vi "Create AI Channel.vi"(8 "error in (no error)":errorcluster, 11 "AI Setting":T1={"Physical Channel"=["6363/ai0", "6363/ai1", "6363/ai2", "6363/ai3"], "Name to assign"=["AI 0", "AI 1", "AI 2", "AI 3"], "minimum value"=0.0, "maximum value"=10.0, "custom scale name"="Motor_speed", "rate"=1000.0, "samples per channel"=1000, "input terminal configuration"=-1, "units"=10348, "sample mode"=10106} {"sample mode" items=["Default"=-1, "RSE"=10083, "NRSE"=10078, "Differential"=10106, "Pseudodifferential"=12529]; "units" items=["Volts"=10348, "From Custom Scale"=10065]; "input terminal configuration" items=["Default"=-1, "RSE"=10083, "NRSE"=10078, "Differential"=10106, "Pseudodifferential"=12529]; "rate" format="%#_13g"; "maximum value" format="%#_13g"; "minimum value" format="%#_13g"}) -> (0 "error out":errorcluster, 3 "task out":refnum<k21>)   [LabVIEW 2016, in "DAQ Hardware.lvlib"]
uses:
  DAQ Hardware.lvlib
  User Interface/AI Channel Setting.ctl
  <vilib>/DAQmx/create/channels.llb/DAQmx Create Channel (AI-Voltage-Basic).vi
  <vilib>/DAQmx/configure/timing.llb/DAQmx Timing (Sample Clock).vi
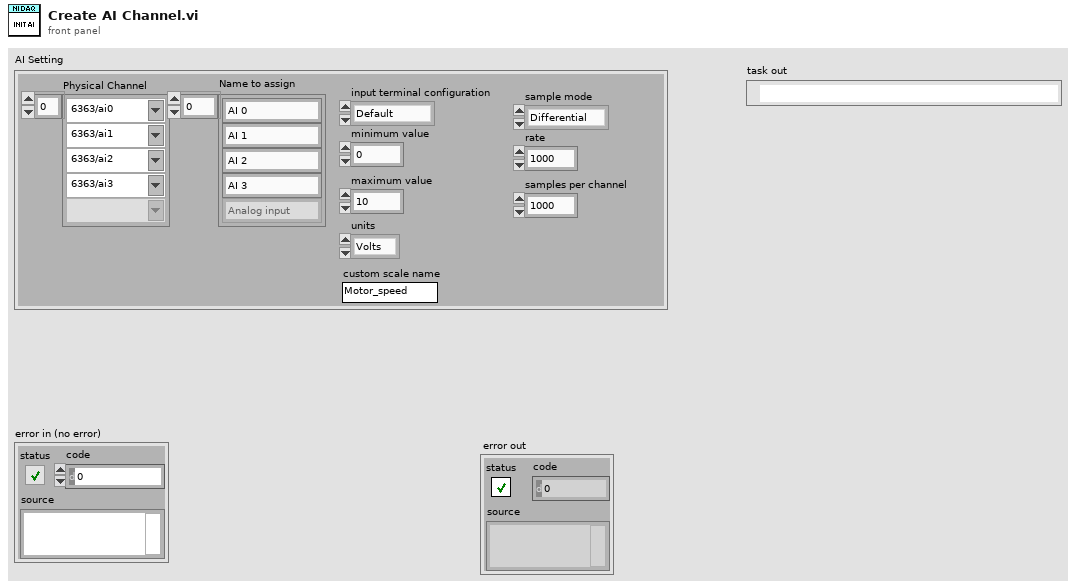
[diagram p1: front panel]
types:
  T1 = typedef "DAQ Hardware.lvlib/AI Channel Setting.ctl" = cluster{"Physical Channel":string[], "Name to assign":string[], "minimum value":dbl, "maximum value":dbl, "custom scale name":string, "rate":dbl, "samples per channel":i32, "input terminal configuration":i32, "units":i32, "sample mode":i32}
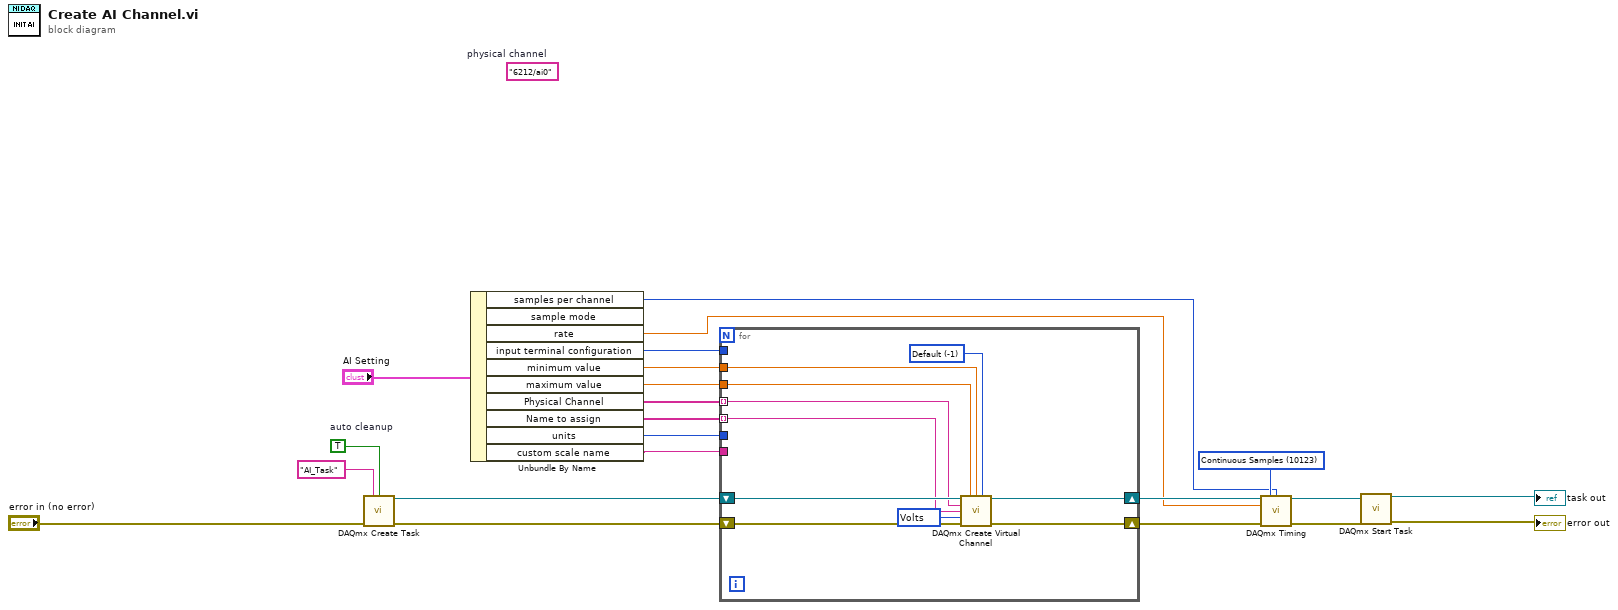
[diagram p0: block diagram]
diagram:
  w2 = 10123 items=["Finite Samples"=10178, "Continuous Samples"=10123, "Hardware Timed Single Point"=12522] ("sample mode")
  w13 = TRUE  # auto cleanup
  (unwired) "6212/ai0"  # physical channel
  n1 = call <vilib>:"DAQmx Create Task.vi"("new task name"="AI_Task", "auto cleanup"=w13, "error in"="error in (no error)") -> ("task out"=w21:refnum<k21>, "error out"=w20:errorcluster)  [unwired: 11 in]
  n2 = Unbundle By Name("AI Setting") -> ("samples per channel"=w1:i32, "rate"=w4:dbl, "input terminal configuration"=w9:i32, "minimum value"=w8:dbl, "maximum value"=w7:dbl, "Physical Channel"=w11:string[], "Name to assign"=w10:string[], "units"=w6:i32, "custom scale name"=w5:string)  [unwired: 1 out]
  n3 = for {
    shift-right: [w32] -> w18
    shift-left: w21 -> [w30]
    shift-right: [w31] -> w19
    shift-left: w20 -> [w29]
    tunnel: w11 -> [w28] mode=indexing
    tunnel: w10 -> [w25] mode=indexing
    tunnel: w9 -> [_]
    tunnel: w8 -> [w27]
    tunnel: w7 -> [w26]
    tunnel: w6 -> [_]
    tunnel: w5 -> [_]
    w23 = 10348 items=["Volts"=10348, "From Custom Scale"=10065] ("units")
    w24 = -1 items=["Default"=-1, "RSE"=10083, "NRSE"=10078, "Differential"=10106, "Pseudodifferential"=12529] ("input terminal configuration")
    n4 = call-poly <vilib>:"DAQmx Create Virtual Channel.vi"("task in"=w30, "maximum value"=w26, "minimum value"=w27, "input terminal configuration"=w24, "physical channels"=w28, "name to assign"=w25, "units"=w23, "error in"=w29) -> ("task out"=w32:refnum<k21>, "error out"=w31:errorcluster)  [unwired: 6 in]
  }
  n5 = call-poly <vilib>:"DAQmx Timing.vi"("task/channels in"=w18, "sample mode"=w2, "samples per channel"=w1, "rate"=w4, "error in"=w19) -> ("task out"=w17:refnum<k21>, "error out"=w16:errorcluster)  [unwired: 9 in]
  n6 = call <vilib>:"DAQmx Start Task.vi"("task/channels in"=w17, "error in"=w16) -> ("task out"=→"task out":refnum<k21>, "error out"=→"error out":errorcluster)  [unwired: 12 in]
